vi "add vi object.vi"(5 "Ring in":refnum<vi>, 8 "error in (no error)":errorcluster, 10 "Add Object Argument":T1, 11 "Data Cluster in":T2) -> (0 "error out":errorcluster, 1 "Result":string, 2 "object_id":i32, 3 "Data Cluster out":T2)   [LabVIEW 2025, in "Scripting Server.lvlib"]
uses:
  Scripting Server.lvlib
  Module Data--cluster.ctl
  Add Object Argument--cluster.ctl
  Add Object (Reply Payload)--cluster.ctl
  <vilib>/Utility/miscctls.llb/LVPointTypeDef.ctl
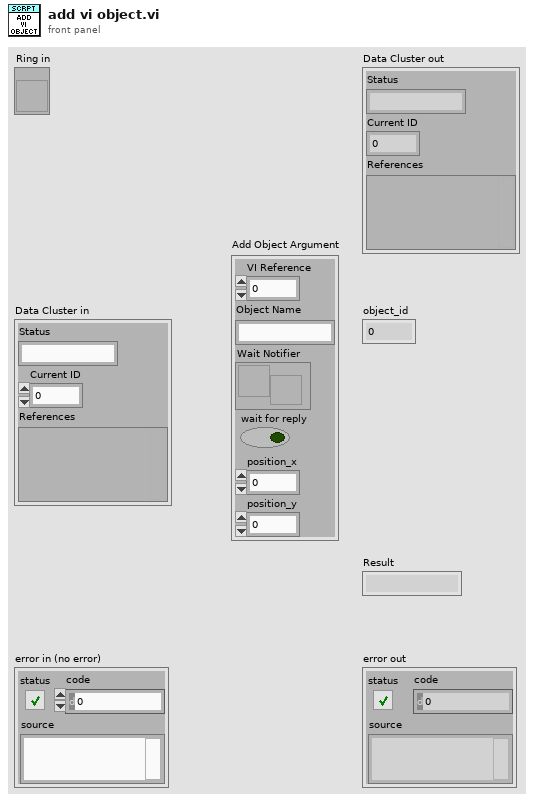
[diagram p1: front panel]
types:
  T1 = typedef "Scripting Server.lvlib/Add Object Argument--cluster.ctl" = cluster{"VI Reference":i32, "Object Name":string, "Wait Notifier":refnum<notifier>, "wait for reply":bool, "position_x":i32, "position_y":i32}
  T2 = typedef "Scripting Server.lvlib/Module Data--cluster.ctl" = cluster{"Status":string, "Current ID":i32, "References":variant}
  T3 = typedef "LVPointTypeDef.ctl" = cluster{"Horizontal":i16, "Vertical":i16}
  T4 = typedef "LVStringsAndValuesArrayTypeDef_I32.ctl" = cluster{"String":string, "Value":i32}[]
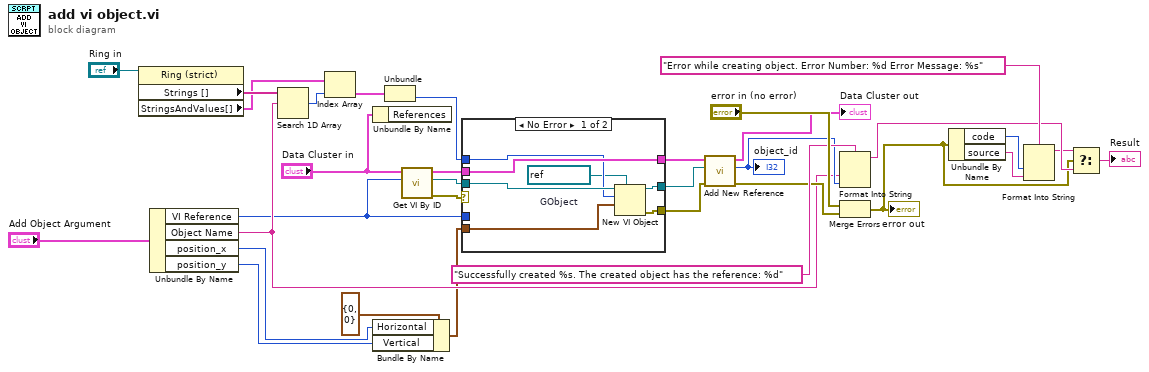
[diagram p0: block diagram]
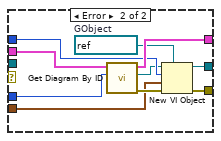
[diagram p2: hidden frame]
diagram:
  n1 = property on="Property Node" class="Ring (strict)"(reference="Ring in") -> ("Strings []"=w30:string[], "StringsAndValues[]"=w29:T4)  [unwired: 1 in, 2 out]
  n2 = Unbundle By Name("Add Object Argument") -> ("VI Reference"=w7:i32, "Object Name"=w11:string, "position_x"=w10:i32, "position_y"=w9:i32)
  n3 = Search 1D Array(1D array=w30, element=w11) -> (index of element=w28:i32)  [unwired: 1 in]
  n4 = Index Array(array=w29, index=w28) -> (element=w31:cluster{"String":string, "Value":i32})
  n5 = Unbundle By Name("Data Cluster in") -> ()  [unwired: 1 out]
  n6 = Bundle By Name(cluster=T3 {"Horizontal"=0, "Vertical"=0} ("location"), "Horizontal"=w10, "Vertical"=w9) -> (w4:T3)
  n7 = Unbundle(w31) -> ("Value"=w3:i32)  [unwired: 1 out]
  n8 = call "Get VI By ID.vi"("ID"=w7, "Data Cluster in"="Data Cluster in") -> ("error out"=w6:errorcluster, "VI Reference"=w5:refnum<vi>, "Data Cluster out"=w8:T2)  [unwired: 7 in]
  n9 = case shown="No Error" w6 {
    tunnel: [w38 w49] -> w13
    tunnel: w7 -> [_ w48]
    tunnel: w8 -> [w38 w47]
    tunnel: w5 -> [w37 _]
    tunnel: w4 -> [w34 w45]
    tunnel: w3 -> [w35 w44]
    tunnel: [w39 w42] -> w2
    tunnel: [w36 w41] -> w1
    frame No Error {
      w33 = refnum<vi> refnum  # GObject
      n10 = New VI Object(vi object class=w33, owner refnum=w37, style=w35, position/next to=w34) -> (object refnum=w36:refnum<vi>, 0:w39:errorcluster)  [unwired: 4 in]
    }
    frame Error {
      w40 = refnum<vi> refnum  # GObject
      n11 = call "Get Diagram By ID.vi"("ID"=w48, "Data Cluster in"=w47) -> ("error out"=w46:errorcluster, "Diagram"=w43:refnum<vi>, "Data Cluster out"=w49:T2)  [unwired: 7 in]
      n12 = New VI Object(vi object class=w40, owner refnum=w43, style=w44, position/next to=w45, 8:w46) -> (object refnum=w41:refnum<vi>, 0:w42:errorcluster)  [unwired: 3 in]
    }
  }
  n13 = call "Add New Reference.vi"("error in (no error)"=w2, "Variant"=w1, "Data Cluster in"=w13) -> ("error out"=w17:errorcluster, "new reference"=w15:i32, "Data Cluster out 2"=→"Data Cluster out":T2)  [unwired: 6 in]
  "object_id" <- w15
  n14 = Format Into String(format string="Successfully created %s. The created object has the reference: %d", w11, w15) -> (resulting string=w23:string)  [unwired: 2 in, 1 out]
  n15 = Merge Errors("error in (no error)", w17) -> (w20:errorcluster)
  "error out" <- w20
  n16 = Unbundle By Name(w20) -> ("code"=w19:i32, "source"=w18:string)
  n17 = Format Into String(format string="Error while creating object. Error Number: %d Error Message: %s" ("f"), w19, w18) -> (resulting string=w21:string)  [unwired: 2 in, 1 out]
  n18 = Select(t=w21, s=w20, f=w23) -> (s? t:f=→"Result":string)
